vi "Close Plugin SubPanel.vi"(8 "error in (no error)":errorcluster, 10 "gRPC Port":i32, 11 "CIF_UI in":refnum<class "CIF_Manager_UI.lvclass">) -> (0 "error out":errorcluster, 3 "CIF_UI out":refnum<class "CIF_Manager_UI.lvclass">)   [LabVIEW 2021, in "CIF_Manager_UI.lvclass"]
uses:
  CIF_Manager_UI.lvclass
  C:/Program Files/National Instruments/LabVIEW 2021/vi.lib/CIF Foundation/CIF Core/CIFUI/CIF_UI.lvclass
  <vilib>/CIF Foundation/CIF Core/CIFUI/CIF_UI.lvclass/CIF_UI.ctl
  <vilib>/CIF Foundation/CIF Core/CIFUI/Accessors/Read Plugin Subpanel Map.vi
  <vilib>/CIF Foundation/CIF Core/CIFUI/Accessors/Write Plugin Subpanel Map.vi
  CIF_Manager_UI.lvclass/CIF_Manager_UI.ctl
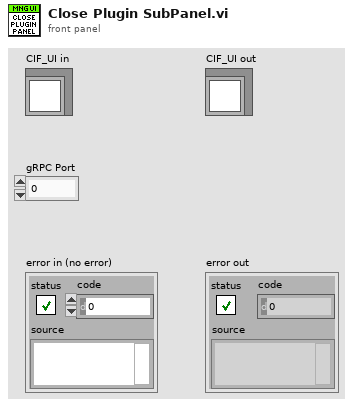
[diagram p1: front panel]
types:
  T1 = typedef "CIF_UI.lvclass/Plugin Subpanel Map.ctl" = map{i32, T2}
  T2 = typedef "CIF_UI.lvclass/Subpanel Data.ctl" = cluster{"VI Reference":refnum<vi>, "Plugin Subpanel Events":T3}
  T3 = typedef "CIF_UI.lvclass/Plugin Subpanel Events.ctl" = cluster{"Plugin Shutdown":refnum<user-event>}
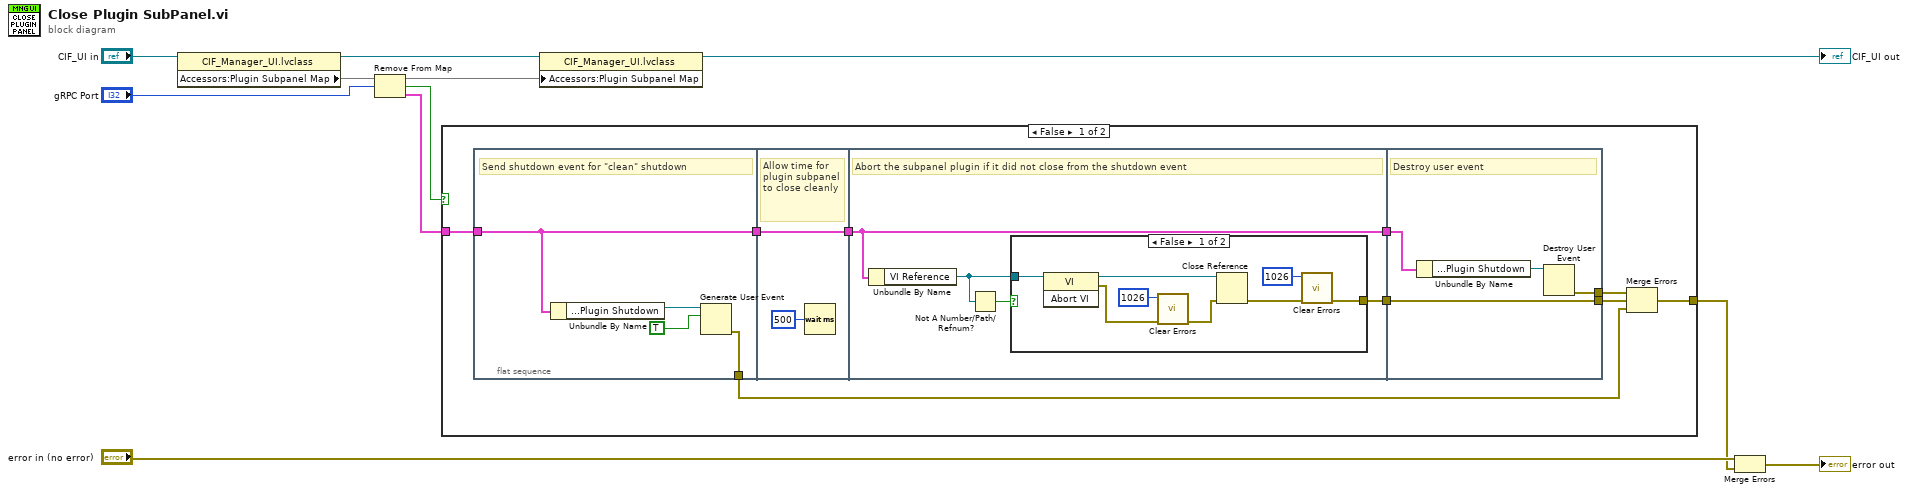
[diagram p0: block diagram]
diagram:
  n1 = property class="CIF_Manager_UI.lvclass"(reference="CIF_UI in") -> (reference out=w2:refnum<class "CIF_Manager_UI.lvclass">, "Accessors:Plugin Subpanel Map"=w4:T1)  [unwired: 1 in, 1 out]
  n2 = Remove From Map(10:"gRPC Port", 11:w4) -> (1:w7:T2, 2:w6:bool, 3:w3:T1)
  n3 = case shown="False" w6 {
    tunnel: [w12 _] -> w10
    tunnel: w7 -> [w20 _]
    frame False {
      n4 = flat-sequence {
        tunnel: w20 -> [w22]
        tunnel: [w22] -> w18
        tunnel: [w21] -> w13
        tunnel: [w26] -> w19
        tunnel: w18 -> [w26]
        tunnel: w19 -> [w27]
        tunnel: [w30] -> w17
        tunnel: [w27] -> w16
        tunnel: [w42] -> w14
        tunnel: w17 -> [w42]
        tunnel: w16 -> [w41]
        tunnel: [w39] -> w15
        frame #0 {
          # "Send shutdown event for \"clean\" shutdown"
          n5 = Unbundle By Name(w22) -> ("Plugin Subpanel Events.Plugin Shutdown"=w24:refnum<user-event>)
          n6 = Generate User Event(user event=w24, event data cluster=TRUE ("event data")) -> (error out=w21:errorcluster)  [unwired: 2 in, 1 out]
        }
        frame #1 {
          # "Allow time for plugin subpanel to close cleanly"
          n7 = Wait (ms)(milliseconds to wait=u32 500) -> ()  [unwired: 1 out]
        }
        frame #2 {
          # "Abort the subpanel plugin if it did not close from the shutdown event"
          n8 = Unbundle By Name(w27) -> ("VI Reference"=w28:refnum<vi>)
          n9 = Not A Number/Path/Refnum?(number/path/refnum=w28) -> (NaN/Path/Refnum?=w29:bool)
          n10 = case shown="False" w29 {
            tunnel: w28 -> [w38 _]
            tunnel: [w31 _] -> w30
            frame False {
              n11 = invoke class="VI" method="Abort VI"(reference=w38) -> (reference out=w37:refnum<vi>, error out=w35:errorcluster)  [unwired: 2 in, 1 out]
              n12 = call <vilib>:"Clear Errors.vi"("error in (no error)"=w35, "specific error code to clear (0: all)"=1026) -> ("error out"=w34:errorcluster)  [unwired: 4 in, 1 out]
              n13 = Close Reference(reference=w37, error in (no error)=w34) -> (error out=w32:errorcluster)
              n14 = call <vilib>:"Clear Errors.vi"("error in (no error)"=w32, "specific error code to clear (0: all)"=1026) -> ("error out"=w31:errorcluster)  [unwired: 4 in, 1 out]
            }
            frame True {
            }
          }
        }
        frame #3 {
          # "Destroy user event"
          n15 = Unbundle By Name(w41) -> ("Plugin Subpanel Events.Plugin Shutdown"=w40:refnum<user-event>)
          n16 = Destroy User Event(user event=w40) -> (error out=w39:errorcluster)  [unwired: 1 in]
        }
      }
      n17 = Merge Errors(w15, w14, w13) -> (w12:errorcluster)
    }
    frame True {
    }
  }
  n18 = property class="CIF_Manager_UI.lvclass"(reference=w2, "Accessors:Plugin Subpanel Map"=w3) -> (reference out=→"CIF_UI out":refnum<class "CIF_Manager_UI.lvclass">)  [unwired: 1 in, 1 out]
  n19 = Merge Errors("error in (no error)", w10) -> (→"error out":errorcluster)
